vi "Sampler Example.vi"() -> ()   [LabVIEW 2011]
uses:
  C:/Program Files/Metrohm Autolab/Autolab SDK 1.10/EcoChemie.Autolab.Sdk.dll
  EcoChemie.Autolab.Sdk.dll
panel:
  out "error out":errorcluster
  in  "stop":bool
  out "IsConnected":bool
  in  "Hardware Setup File":path
  in  "Embedded Exe File":path
  out "Value":dbl
  in  "Signal List":string(combo)
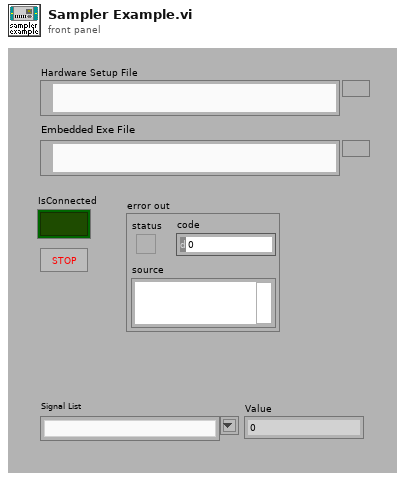
[diagram p1: front panel]
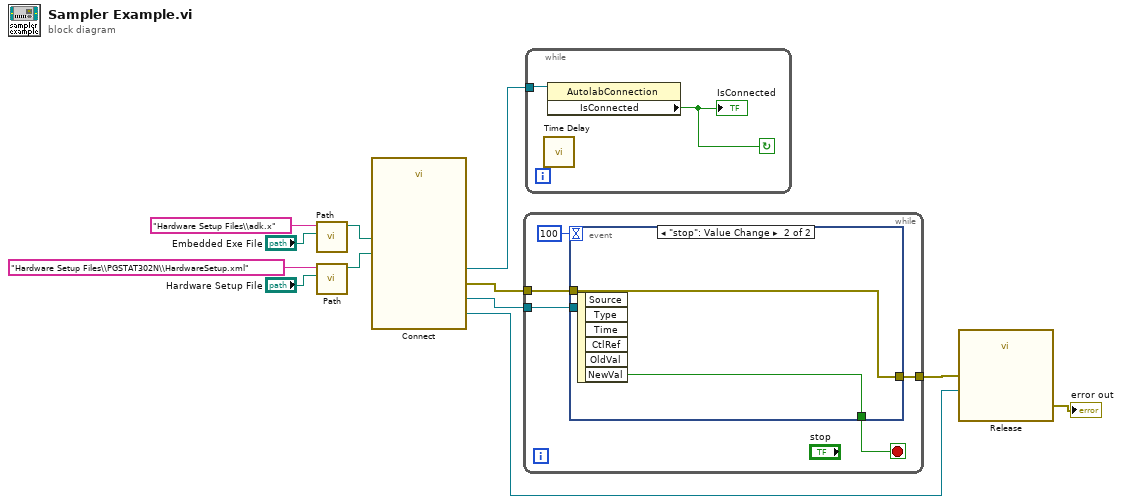
[diagram p0: block diagram]
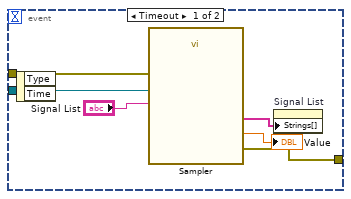
[diagram p2: hidden frame]
diagram:
  n1 = call "Path.vi"("File"="Embedded Exe File", "name or relative path"="Hardware Setup Files\\adk.x") -> ("appended path"=w2:path)  [unwired: 9 in]
  n2 = call "Path.vi"("File"="Hardware Setup File", "name or relative path"="Hardware Setup Files\\PGSTAT302N\\HardwareSetup.xml") -> ("appended path"=w1:path)  [unwired: 9 in]
  n3 = call "Connect.vi"("Embedded Exe File"=w2, "Hardware Setup File"=w1) -> ("Sampler"=w8:refnum<k24>, "AutolabConnection"=w10:refnum<k24>, "instrument"=w7:refnum<k24>, "error out"=w9:errorcluster)  [unwired: 6 in, 4 out]
  n4 = while {
    tunnel: w9 -> [w17]
    tunnel: w8 -> [w16]
    tunnel: [w15] -> w12
    stop <- w13 stop-if-true
    n5 = event shown="[1] \"stop\": Value Change" {
      selector: _ -> [_ _]
      dyn-events: _ -> [_ _]
      timeout: 100 -> [_ _]
      tunnel: w17 -> [w23 w24]
      tunnel: w16 -> [w22 _]
      tunnel: [w18 w24] -> w15
      tunnel: [_ w25] -> w13
      event Timeout {
        n6 = event-data() -> ()  [unwired: 1 in, 2 out]
        n7 = call "Sampler.vi"("error in (no error)"=w23, "Signal List"="Signal List", "Sampler"=w22) -> ("error out"=w18:errorcluster, "Signal Value"=→"Value":dbl, "GetSignals"=w20:string[])  [unwired: 6 in]
        n8 = property on="Signal List" class="CmbBox"("Strings[]"=w20) -> ()  [unwired: 2 in, 2 out]
      }
      event "stop": Value Change {
        n9 = event-data() -> ("NewVal"=w25:bool)  [unwired: 1 in, 5 out]
      }
    }
  }
  n10 = while {
    tunnel: w10 -> [w27]
    stop <- w26 continue-if-true
    n11 = call "Time Delay"() -> ()  [unwired: 11 in, 1 out]
    n12 = property class="AutolabConnection"(reference=w27) -> ("IsConnected"=w26:bool)  [unwired: 1 in, 2 out]
    "IsConnected" <- w26
  }
  n13 = call "Release.vi"("error in (no error)"=w12, "Instrument"=w7) -> ("error out"=→"error out":errorcluster)  [unwired: 9 in]
